vi "Close.vi"(8 "error in (no error)":errorcluster, 11 "Dali_usb_tridonics in":refnum<class "Dali_usb_tridonics.lvclass">) -> (0 "error out":errorcluster, 3 "Dali_usb_tridonics out":refnum<class "Dali_usb_tridonics.lvclass">)   [LabVIEW 2014, in "Driver_interaction.lvlib" / "Dali_usb_tridonics.lvclass"]
uses:
  Dali_usb_tridonics.lvclass
  Dali_usb_tridonics.lvclass/Dali_usb_tridonics.ctl
  _Driver_interaction/_Driver_interaction.lvclass
  Vendor/Dali_usb.lvlib
panel:
  out "close_response":i32
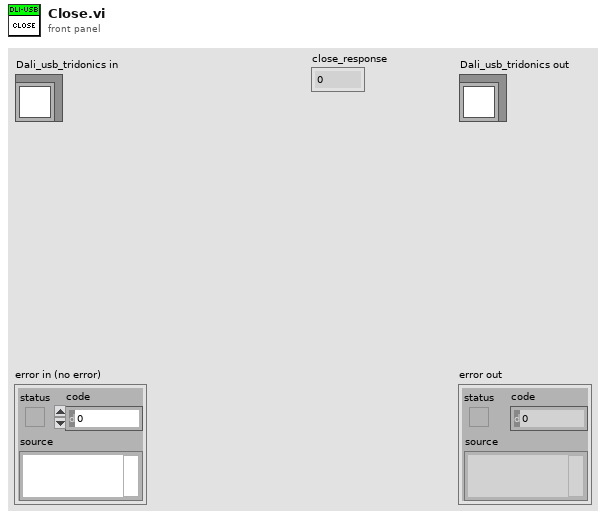
[diagram p1: front panel]
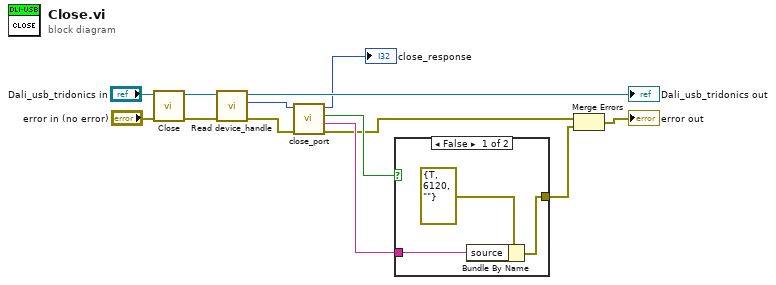
[diagram p0: block diagram]
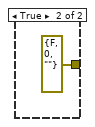
[diagram p2: hidden frame]
diagram:
  n1 = call-parent "Close.vi"("error in (no error)"="error in (no error)", "_Driver_interaction in"="Dali_usb_tridonics in") -> ("error out"=w9:errorcluster, "_Driver_interaction out"=w11:refnum<class "Dali_usb_tridonics.lvclass">)  [unwired: 8 in]
  n2 = call "Read device_handle.vi"("error in (no error)"=w9, "Dali_usb_tridonics in"=w11) -> ("error out"=w4:errorcluster, "device_handle"=w8:i32, "Dali_usb_tridonics out"=→"Dali_usb_tridonics out":refnum<class "Dali_usb_tridonics.lvclass">)  [unwired: 7 in]
  n3 = call "close_port.vi"("error in (no error)"=w4, "device_handle"=w8) -> ("error out"=w2:errorcluster, "failstring"=w6:string, "closed"=w7:bool, "close_response"=→"close_response":i32)  [unwired: 6 in]
  n4 = case shown="False" w7 {
    tunnel: w6 -> [w15 _]
    tunnel: [w14 errorcluster {"status"=FALSE, "code"=0, "source"=""} ("error out")] -> w3
    frame False {
      n5 = Bundle By Name(cluster=errorcluster {"status"=TRUE, "code"=6120, "source"=""} ("error out"), "source"=w15) -> (w14:errorcluster)
    }
    frame True {
    }
  }
  n6 = Merge Errors(w2, w3) -> (→"error out":errorcluster)
